vi "Send Command.vi"(8 "error in (no error)":errorcluster, 9 "Data":variant, 10 "Command":T1, 11 "QTab Class in":refnum<class "QTab Class.lvclass">) -> (0 "error out":errorcluster, 3 "QTab Class out":refnum<class "QTab Class.lvclass">)   [LabVIEW 2020, in "QTab.lvlib" / "QTab Class.lvclass"]
uses:
  QTab Class.lvclass
  Command.ctl
  Command Data.ctl
  QTab Class.lvclass/QTab Class.ctl
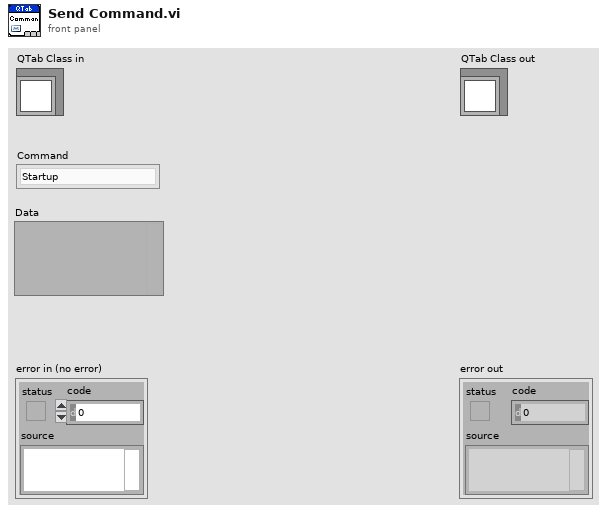
[diagram p1: front panel]
types:
  T1 = typedef "QTab.lvlib/QTab Class.lvclass/Command.ctl" = enum16{"Startup", "Add Page", "Close All Page", "Set Page Attribute", "Pop-out", "Merage", "Insert", "Stop"}
  T2 = typedef "QTab.lvlib/QTab Class.lvclass/Command Data.ctl" = cluster{"Command":T1, "Data":variant}
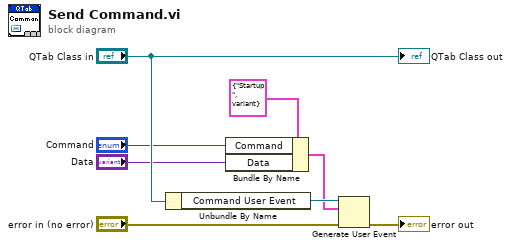
[diagram p0: block diagram]
diagram:
  n1 = Unbundle By Name("QTab Class in") -> ("Command User Event"=w8:refnum<user-event>)
  n2 = Bundle By Name(cluster=T2 {"Command"=enum."Startup", "Data"=variant} ("Command Data"), "Command"="Command", "Data"="Data") -> (w7:T2)
  n3 = Generate User Event(user event=w8, event data cluster=w7, error in="error in (no error)") -> (error out=→"error out":errorcluster)  [unwired: 1 in, 1 out]
  "QTab Class out" <- "QTab Class in"
